vi "VIListReload.vi"(8 "error in (no error)":errorcluster, 11 "VI List in":refnum<vi>) -> (3 "VI List out":refnum<vi>)   [LabVIEW 2019, in "VIPropertyPicker.lvlib"]
uses:
  VIPropertyPicker.lvlib
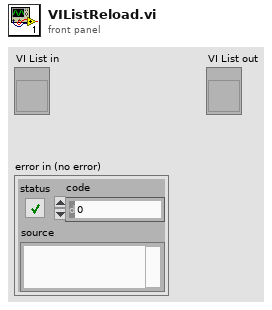
[diagram p1: front panel]
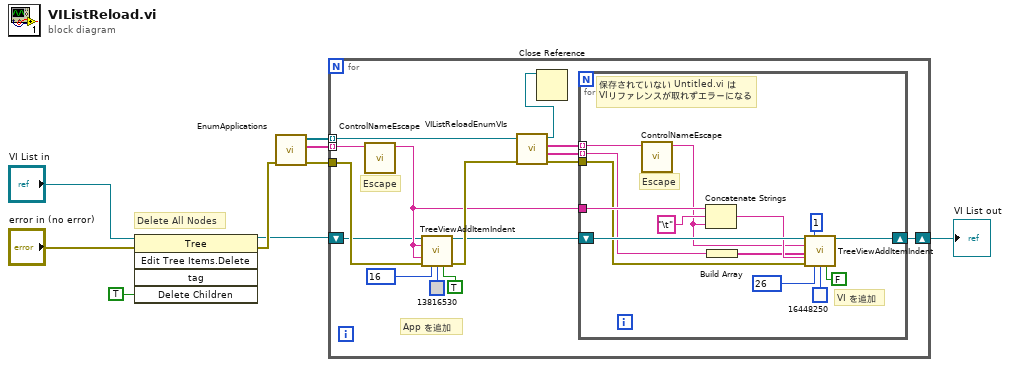
[diagram p0: block diagram]
diagram:
  # "Delete All Nodes"
  n1 = invoke class="Tree" method="Edit Tree Items.Delete"(reference="VI List in", error in="error in (no error)", "Delete Children"=TRUE ("Delete Children?")) -> (reference out=w7:refnum<vi>, error out=w8:errorcluster)  [unwired: 2 in, 3 out]
  n2 = call "EnumApplications.vi"("error in (no error)"=w8) -> ("error out"=w5:errorcluster, "Application Names"=w9:string[], "Application References"=w4:refnum<vi>[])  [unwired: 8 in]
  n3 = for {
    tunnel: w4 -> [w16] mode=indexing
    tunnel: w9 -> [w19] mode=indexing
    shift-right: [w17] -> w1
    shift-left: w7 -> [w13]
    tunnel: w5 -> [w18]
    # "Escape"
    # "App を追加"
    n4 = call "ControlNameEscape.vi"("label"=w19) -> ("escaped string"=w14:string)  [unwired: 10 in]
    n5 = call "TreeViewAddItemIndent.vi"("TreeControl in"=w13, "Left Cell String"=w14, "Tag"=w14, "error in (no error)"=w18, "Symbol Index"=16, "Background Color"=u32 13816530, "Bold Font"=TRUE) -> ("TreeControl out"=w22:refnum<vi>, "error out"=w24:errorcluster)  [unwired: 6 in, 1 out]
    n6 = call "VIListReloadEnumVIs.vi"("error in (no error)"=w24, "Application in"=w16) -> ("error out"=w20:errorcluster, "Paths"=w11:string[], "VI Tags"=w15:string[], "Application out"=w10:refnum<vi>)  [unwired: 6 in]
    n7 = Close Reference(reference=w10) -> ()  [unwired: 1 in, 1 out]
    n8 = for {
      tunnel: w15 -> [w34] mode=indexing
      tunnel: w14 -> [w37]
      shift-right: [w29] -> w17
      shift-left: w22 -> [w38]
      tunnel: w20 -> [w28]
      tunnel: w11 -> [w25] mode=indexing
      # "VI を追加"
      # "Escape"
      # "保存されていない Untitled.vi は\nVIリファレンスが取れずエラーになる"
      n9 = call "ControlNameEscape.vi"("label"=w34) -> ("escaped string"=w33:string)  [unwired: 10 in]
      n10 = Concatenate Strings(w37, "\t" ("string"), w33) -> (w35:string)
      n11 = Build Array(w25) -> (w26:string[])
      n12 = call "TreeViewAddItemIndent.vi"("TreeControl in"=w38, "Indentation"=1, "Left Cell String"=w33, "Child Text"=w26, "Tag"=w35, "error in (no error)"=w28, "Symbol Index"=26, "Background Color"=u32 16448250, "Bold Font"=FALSE) -> ("TreeControl out"=w29:refnum<vi>)  [unwired: 4 in, 2 out]
    }
  }
  "VI List out" <- w1
